vi "Error Query.vi"(8 "error in (no error)":errorcluster, 11 "VISA resource name":refnum<visa-resource-name>) -> (0 "error out":errorcluster, 1 "Error Message":string, 2 "Error Code":i32[](array[numeric]), 3 "VISA resource name out":refnum<visa-resource-name>)   [LabVIEW 2014, in "Agilent PSG MXG Series.lvlib"]
doc: "Queries the instrument for any errors in the instrument's error queue. It will continue to read errors until all errors have been read from the instrument. Any errors will be returned in the <B>error out</B> control.\n\n<B>Note:</B>\nThis VI is called automatically by most driver VIs so it is not usually necessary to call this in an application."
uses:
  Agilent PSG MXG Series.lvlib
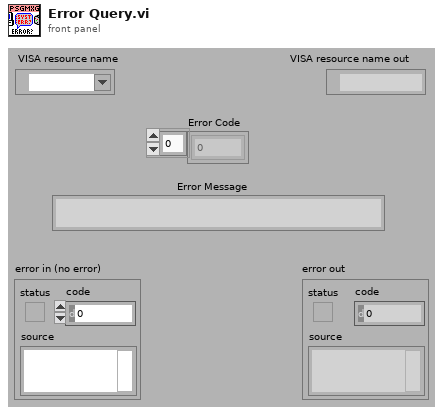
[diagram p1: front panel]
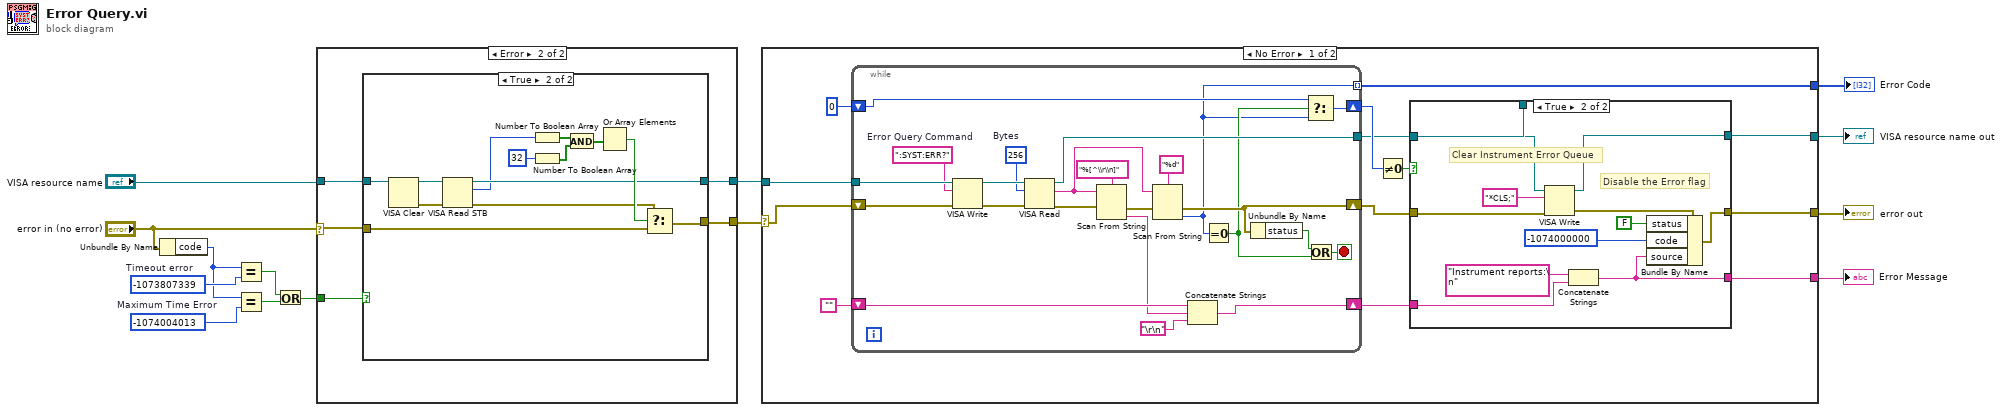
[diagram p0: block diagram]
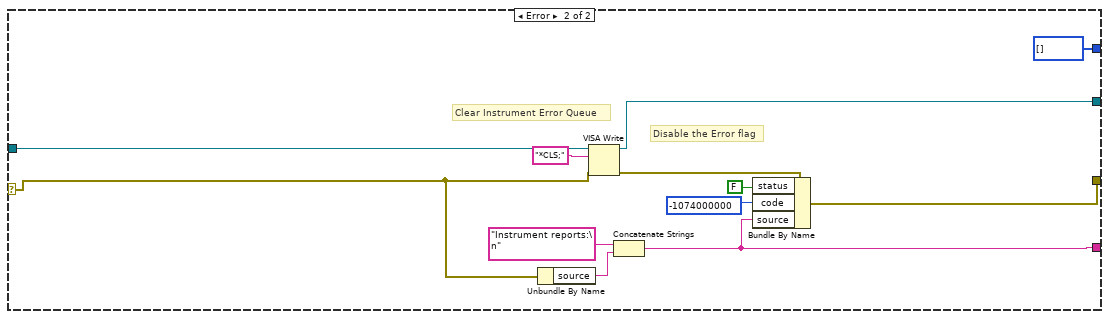
[diagram p5: hidden frame]
diagram:
  w5 = -1074004013  # Maximum Time Error
  w7 = -1073807339  # Timeout error
  n1 = Unbundle By Name("error in (no error)") -> ("code"=w6:i32)
  n2 = Equal?(x=w6, y=w7) -> (x = y?=w3:bool)
  n3 = Equal?(x=w6, y=w5) -> (x = y?=w4:bool)
  n4 = Or(x=w3, y=w4) -> (x .or. y?=w2:bool)
  n5 = case shown="Error" "error in (no error)" {
    selector: "error in (no error)" -> [w15 w19]
    tunnel: "VISA resource name" -> [w16 w21]
    tunnel: [w16 w20] -> w9
    tunnel: [w15 w18] -> w10
    tunnel: w2 -> [_ w17]
    frame No Error {
    }
    frame Error {
      n6 = case shown="True" w17 {
        tunnel: w21 -> [w23 w29]
        tunnel: [w23 w26] -> w20
        tunnel: w19 -> [w22 w32]
        tunnel: [w22 w31] -> w18
        frame False {
        }
        frame True {
          n7 = VISA Clear(VISA resource name=w29) -> (VISA resource name out=w28:refnum<visa-resource-name>, error out=w27:errorcluster)  [unwired: 1 in]
          n8 = VISA Read STB(8:w27, 11:w28) -> (0:w25:errorcluster, 2:w24:u16, 3:w26:refnum<visa-resource-name>)
          n9 = Number To Boolean Array(number=w24) -> (Boolean array=w33:bool[])
          n10 = Number To Boolean Array(number=32) -> (Boolean array=w35:bool[])
          n11 = And(x=w33, y=w35) -> (x .and. y?=w34:bool[])
          n12 = Or Array Elements(Boolean array=w34) -> (logical OR=w30:bool)
          n13 = Select(t=w25, s=w30, f=w32) -> (s? t:f=w31:errorcluster)
        }
      }
    }
  }
  n14 = case shown="No Error" w10 {
    selector: w10 -> [w41 w95]
    tunnel: [w39 w92] -> w14
    tunnel: w9 -> [w49 w93]
    tunnel: [w37 w90] -> w13
    tunnel: [w38 w87] -> w12
    tunnel: [w43 i32[] []] -> w11
    frame No Error {
      n15 = while {
        tunnel: [w86] -> w40
        tunnel: w49 -> [w85]
        shift-right: [w73] -> w44
        shift-left: "" ("Empty String Constant") -> [w76]
        shift-right: [w71] -> w45
        shift-left: 0 -> [w72]
        shift-right: [w69] -> w42
        shift-left: w41 -> [w70]
        tunnel: [w64] -> w43 mode=indexing
        stop <- w79 stop-if-true
        w83 = u32 256  # Bytes
        w81 = ":SYST:ERR?"  # Error Query Command
        n16 = VISA Write(VISA resource name=w85, write buffer=w81, error in (no error)=w70) -> (VISA resource name out=w84:refnum<visa-resource-name>, error out=w82:errorcluster)  [unwired: 1 out]
        n17 = VISA Read(VISA resource name=w84, byte count=w83, error in (no error)=w82) -> (VISA resource name out=w86:refnum<visa-resource-name>, read buffer=w77:string, error out=w68:errorcluster)  [unwired: 1 out]
        n18 = Scan From String(format string="%[^\\r\\n]", input string=w77, error in=w68) -> (error out=w67:errorcluster, output 1=w74:string)  [unwired: 1 in, 3 out]
        n19 = Scan From String(format string="%d", input string=w77, error in=w67) -> (error out=w69:errorcluster, output 1=w64:i32)  [unwired: 1 in, 3 out]
        n20 = Concatenate Strings(w76, w74, "\r\n" ("End of Line Constant")) -> (w73:string)
        n21 = Equal To 0?(x=w64) -> (x = 0?=w65:bool)
        n22 = Unbundle By Name(w69) -> ("status"=w66:bool)
        n23 = Select(t=w72, s=w65, f=w64) -> (s? t:f=w71:i32)
        n24 = Or(x=w66, y=w65) -> (x .or. y?=w79:bool)
      }
      n25 = Not Equal To 0?(x=w45) -> (x != 0?=w46:bool)
      n26 = case shown="True" w46 {
        tunnel: w44 -> [w50 w62]
        tunnel: [w52 w55] -> w37
        tunnel: w42 -> [w52 w61]
        tunnel: w40 -> [_ _]
        tunnel: w40 -> [w51 w59]
        tunnel: [w51 w58] -> w39
        tunnel: [w50 w53] -> w38
        frame False {
        }
        frame True {
          # "Disable the Error flag"
          # "Clear Instrument Error Queue"
          n27 = VISA Write(VISA resource name=w59, write buffer="*CLS;", error in (no error)=w61) -> (VISA resource name out=w58:refnum<visa-resource-name>, error out=w56:errorcluster)  [unwired: 1 out]
          n28 = Concatenate Strings("Instrument reports:\n" ("Source"), w62) -> (w53:string)
          n29 = Bundle By Name(cluster=w56, "status"=FALSE ("show call chain? (False)"), "code"=-1074000000 ("Code"), "source"=w53) -> (w55:errorcluster)
        }
      }
    }
    frame Error {
      # "Disable the Error flag"
      # "Clear Instrument Error Queue"
      n30 = Unbundle By Name(w95) -> ("source"=w94:string)
      n31 = VISA Write(VISA resource name=w93, write buffer="*CLS;", error in (no error)=w95) -> (VISA resource name out=w92:refnum<visa-resource-name>, error out=w91:errorcluster)  [unwired: 1 out]
      n32 = Concatenate Strings("Instrument reports:\n" ("Source"), w94) -> (w87:string)
      n33 = Bundle By Name(cluster=w91, "status"=FALSE ("show call chain? (False)"), "code"=-1074000000 ("Code"), "source"=w87) -> (w90:errorcluster)
    }
  }
  "VISA resource name out" <- w14
  "error out" <- w13
  "Error Message" <- w12
  "Error Code" <- w11
